vi "Delete Group.vi"(8 "error in (no error)":errorcluster, 11 "Group":string) -> (0 "error out":errorcluster)   [LabVIEW 2016, in "CVT.lvlib" / "Current Value Table.lvlib"]
doc: "This VI forms a named group which can be used to later read or write data to that entire group. This has the same functionality as including a set of groups during initialization. Tags can be members of multiple groups without issue."
uses:
  Current Value Table.lvlib
  FGVs/Group Memory Methods.ctl
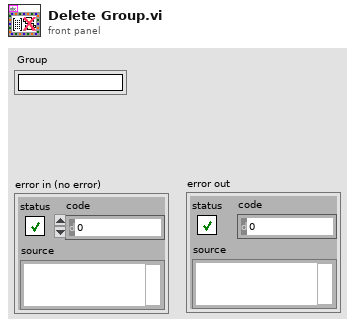
[diagram p1: front panel]
types:
  T1 = typedef "CVT.lvlib/Current Value Table.lvlib/Group Memory Methods.ctl" = enum16{"Clear", "Read Indices in Group", "List Groups", "List Tags by Type", "List Tags", "Delete Group", "Check Group Existence", "Create Group"}
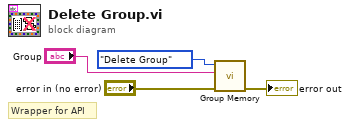
[diagram p0: block diagram]
diagram:
  # "Wrapper for API"
  n1 = call "Group Memory.vi"("error in (no error)"="error in (no error)", "Group"="Group", "Method"=Group_Memory_Methods."Delete Group") -> ("error out"=→"error out":errorcluster)  [unwired: 5 in, 3 out]
